vi "Main CPU Bars Viewer.vi"() -> ()   [LabVIEW 2016]
uses:
  <vilib>/LIEF/Image Editor Handler/Image Editor Handler.lvclass
  <vilib>/LIEF/Image Editor Handler/Image Editor Handler.lvclass/Image Editor Handler.ctl
  <vilib>/LIEF/Image Editor Handler/Read Events.vi
  <vilib>/LIEF/Forms/Shape/Shape.lvclass
  <vilib>/nisyscfg/nisyscfg.lvlib
  <resource>/objmgr/nisysapi.rc
  <resource>/objmgr/motionsysapi.rc
  CPU Bar/CPU Bar.lvclass
  <vilib>/LIEF/Forms/Grid/Grid.lvclass
panel:
  in  "2D Picture":picture
  # "1. Run the VI and wait until the CPU Bars start refreshing\n2. Stop the VI and resize the picture control. Re-run."
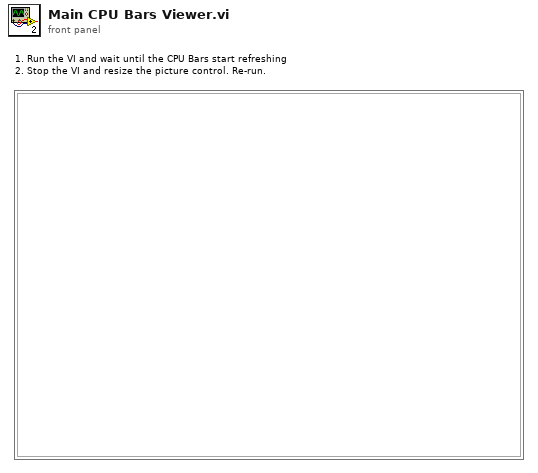
[diagram p1: front panel]
types:
  T1 = typedef "LVBoundsTypeDef.ctl" = cluster{"Width":u32, "Height":u32}
  T2 = typedef "LV Image Editor Framework.lvlib/Image Editor Handler.lvclass/Editor Events.ctl" = cluster{"Stop":refnum<user-event>, "Image Events":cluster{"AddShape":refnum<user-event>, "Paint":refnum<user-event>, "RemoveShape":refnum<user-event>, "RefreshShape ByRef":refnum<user-event>, "ShapePropertyChange":refnum<user-event>, "RemoveShape ByRef":refnum<user-event>}, "RequestShapes":refnum<user-event>, "Custom":refnum<user-event>}
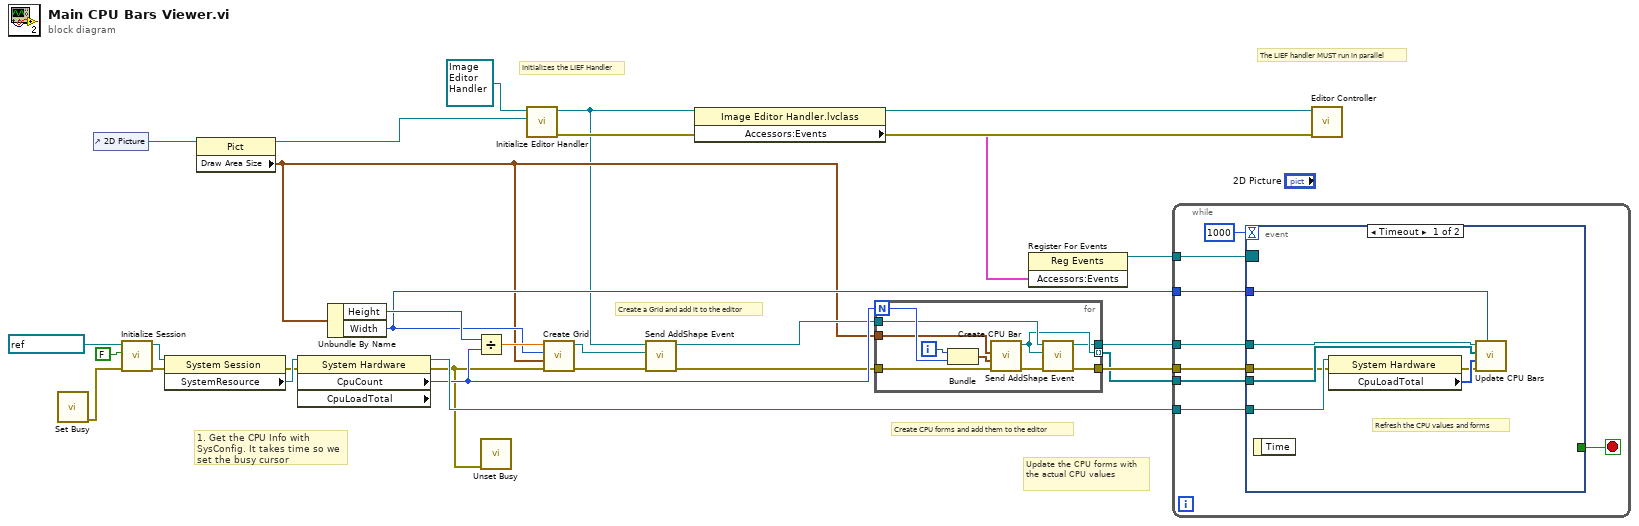
[diagram p0: block diagram]
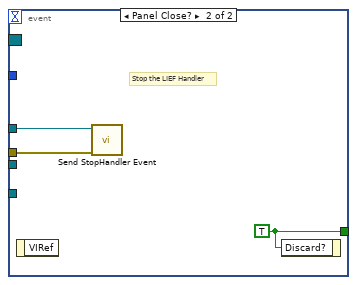
[diagram p2: hidden frame]
diagram:
  # "Update the CPU forms with the actual CPU values"
  # "Create CPU forms and add them to the editor"
  # "Create a Grid and add it to the editor"
  # "The LIEF handler MUST run in parallel"
  # "Initializes the LIEF Handler"
  # "1. Get the CPU Info with SysConfig. It takes time so we set the busy cursor"
  n1 = call <vilib>:"Set Busy.vi"() -> ("error out"=w4:errorcluster)  [unwired: 10 in, 1 out]
  n2 = control-ref of="2D Picture"() -> (w22:refnum<vi>)
  n3 = call <vilib>:"Initialize Session.vi"("error in (no error)"=w4, "Force Property Refresh (T)"=FALSE, "Target (localhost)"=refnum<k21> "localhost") -> ("error out"=w18:errorcluster, "Session out"=w28:refnum<k21>)  [unwired: 7 in]
  n4 = property class="System Session"(reference=w28, error in=w18) -> (error out=w19:errorcluster, "SystemResource"=w23:refnum<k20>)  [unwired: 1 out]
  n5 = property class="Pict"(reference=w22) -> (reference out=w6:refnum<vi>, "Draw Area Size"=w5:T1)  [unwired: 1 in, 1 out]
  n6 = property class="System Hardware" props=["CpuCount", "CpuLoadTotal"](reference=w23, error in=w19) -> (reference out=w17:refnum<k20>, error out=w3:errorcluster, "CpuCount"=w14:i32)  [unwired: 1 out]
  n7 = Unbundle By Name(w5) -> ("Height"=w13:u32, "Width"=w11:u32)
  n8 = Divide(x=w13, y=w14) -> (x/y=w12:dbl)
  n9 = call <vilib>:"Unset Busy.vi"("error in (no error)"=w3) -> ()  [unwired: 10 in, 1 out]
  n10 = call <vilib>:"Initialize Editor Handler.vi"("PictureRef"=w6, "Editor Handler in"=refnum<class "Image Editor Handler.lvclass"> refnum) -> ("error out"=w15:errorcluster, "Editor Handler out"=w2:refnum<class "Image Editor Handler.lvclass">)  [unwired: 8 in]
  n11 = call <vilib>:"Create Grid.vi"("error in (no error)"=w3, "Draw Area"=w5, "Horizontal Step"=w11, "Vertical Step"=w12) -> ("error out"=w8:errorcluster, "Grid Reference"=w9:refnum<data-value>)  [unwired: 6 in]
  n12 = call <vilib>:"Send AddShape Event.vi"("error in (no error)"=w8, "New Shape Reference"=w9, "Editor Handler in"=w2) -> ("error out"=w7:errorcluster, "Editor Handler out"=w10:refnum<class "Image Editor Handler.lvclass">)  [unwired: 7 in]
  n13 = property class="Image Editor Handler.lvclass"(reference=w2) -> ("Accessors:Events"=w1:T2)  [unwired: 1 in, 2 out]
  n14 = for {
    N: w14 -> [w37]
    tunnel: [w34] -> w20 mode=indexing
    tunnel: w10 -> [w35]
    tunnel: [w33] -> w21
    tunnel: w7 -> [w31]
    tunnel: [w30] -> w16
    tunnel: w5 -> [w29]
    i -> [w38]
    n15 = Bundle(w38, w37) -> (w36:cluster{i32, i32})  [unwired: 1 in]
    n16 = call "Create CPU Bar.vi"("error in (no error)"=w31, "CPU Info"=w36, "Draw Area Size"=w29) -> ("error out"=w32:errorcluster, "Shape Reference"=w34:refnum<data-value>)  [unwired: 7 in]
    n17 = call <vilib>:"Send AddShape Event.vi"("error in (no error)"=w32, "New Shape Reference"=w34, "Editor Handler in"=w35) -> ("error out"=w33:errorcluster, "Editor Handler out"=w30:refnum<class "Image Editor Handler.lvclass">)  [unwired: 7 in]
  }
  n18 = register-events(w1) -> (reference out=w25:refnum<event-registration>)  [unwired: 2 in, 1 out]
  n19 = while {
    tunnel: w16 -> [w45]
    tunnel: w25 -> [w44]
    tunnel: w17 -> [w42]
    tunnel: w20 -> [w41]
    tunnel: w11 -> [w40]
    tunnel: w21 -> [w39]
    stop <- w46 stop-if-true
    n20 = event shown="[0] Timeout" {
      selector: w44 -> [_ _]
      dyn-events: _ -> [_ _]
      timeout: 1000 -> [_ _]
      tunnel: [_ w56] -> w46
      tunnel: w45 -> [w52 w55]
      tunnel: w42 -> [w53 _]
      tunnel: w41 -> [w51 _]
      tunnel: w40 -> [w49 _]
      tunnel: w39 -> [w48 w54]
      event Timeout {
        # "Refresh the CPU values and forms"
        n21 = event-data() -> ()  [unwired: 1 in, 1 out]
        n22 = property class="System Hardware"(reference=w53, error in=w48) -> (error out=w47:errorcluster, "CpuLoadTotal"=w50:u32[])  [unwired: 1 out]
        n23 = call "Update CPU Bars.vi"("Width"=w49, "error in (no error)"=w47, "CpuLoadTotal"=w50, "Array in"=w51, "Image Editor Handler in"=w52) -> ()  [unwired: 5 in, 2 out]
      }
      event Panel Close? {
        w56 = TRUE ("Discard?")
        # "Stop the LIEF Handler"
        n24 = event-data() -> ()  [unwired: 1 in, 1 out]
        n25 = call <vilib>:"Send StopHandler Event.vi"("error in (no error)"=w54, "Editor Handler in"=w55) -> ()  [unwired: 8 in, 2 out]
        n26 = event-data("Discard?"=w56) -> ()  [unwired: 1 in, 1 out]
      }
    }
  }
  n27 = call <vilib>:"Editor Controller.vi"("error in (no error)"=w15, "Editor Handler in"=w2) -> ()  [unwired: 8 in, 2 out]
